vi "Spatial Dual Decode Packet 54 (SubVI).vi"(8 "SGL Precision":i16=6, 10 "Packet 54 Bytes In":u8[](array[numeric])) -> (0 "Channel Data Type":string[](array[string])=["Float", "Float", "Float"], 1 "Channel Units":string[](array[string])=["m/s/s", "m/s/s", "m/s/s"], 2 "Data":string[](array[string]), 3 "Channel Names":string[](array[string])=["Acc X", "Acc Y", "Acc Z"], 4 "Packet 54 Decoded Data Cluster":cluster{"Geoid Height":sgl})   [LabVIEW 2019, in "SpatialDual_Parsers.lvlib"]
uses:
  SpatialDual_Parsers.lvlib
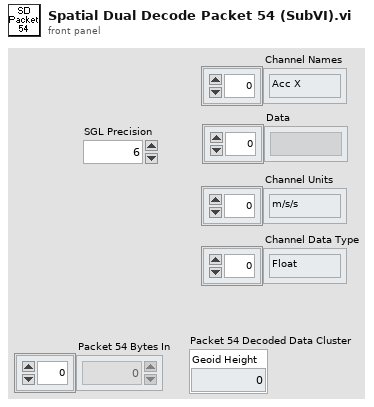
[diagram p1: front panel]
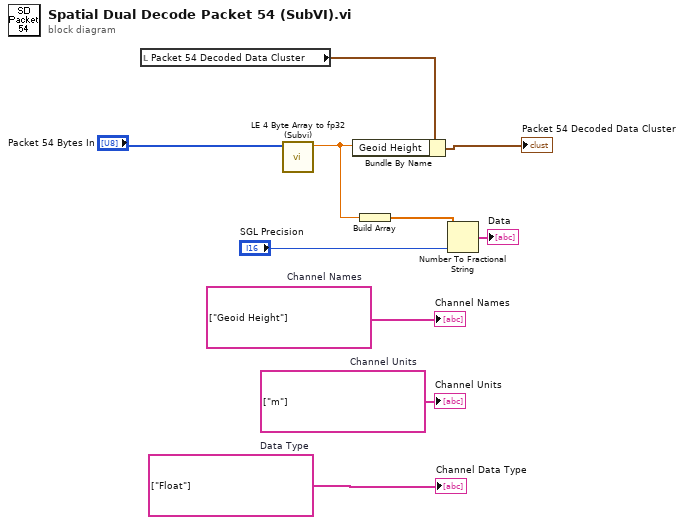
[diagram p0: block diagram]
diagram:
  w2 = string[] ["Float"]  # Data Type
  w3 = string[] ["Geoid Height"]  # Channel Names
  w4 = string[] ["m"]  # Channel Units
  n1 = local read "Packet 54 Decoded Data Cluster"() -> (w10:cluster{"Geoid Height":sgl})
  n2 = call "LE 4 Byte Array to fp32 (Subvi).vi"("4 Bytes in"="Packet 54 Bytes In") -> ("fp32 Out"=w8:sgl)  [unwired: 8 in]
  n3 = Bundle By Name(cluster=w10, "Geoid Height"=w8) -> (→"Packet 54 Decoded Data Cluster":cluster{"Geoid Height":sgl})
  n4 = Build Array(w8) -> (w7:sgl[])
  n5 = Number To Fractional String(number=w7, precision (6)="SGL Precision") -> (F-format string=→"Data":string[])  [unwired: 2 in]
  "Channel Names" <- w3
  "Channel Units" <- w4
  "Channel Data Type" <- w2
